vi "test1.vi"() -> ()   [LabVIEW 2014]
uses:
  <vilib>/Utility/sysdir.llb/System Directory Type.ctl
panel:
  in  "정규식":string
  out "이후 부분 문자열":string
  out "텍스트 2":string
  in  "오프셋(0)":i32=34
  in  "정규식 2":string
  out "이전 부분 문자열":string
  out "텍스트":string
  in  "오프셋(0) 2":i32=4
  out "연결된 문자열":string
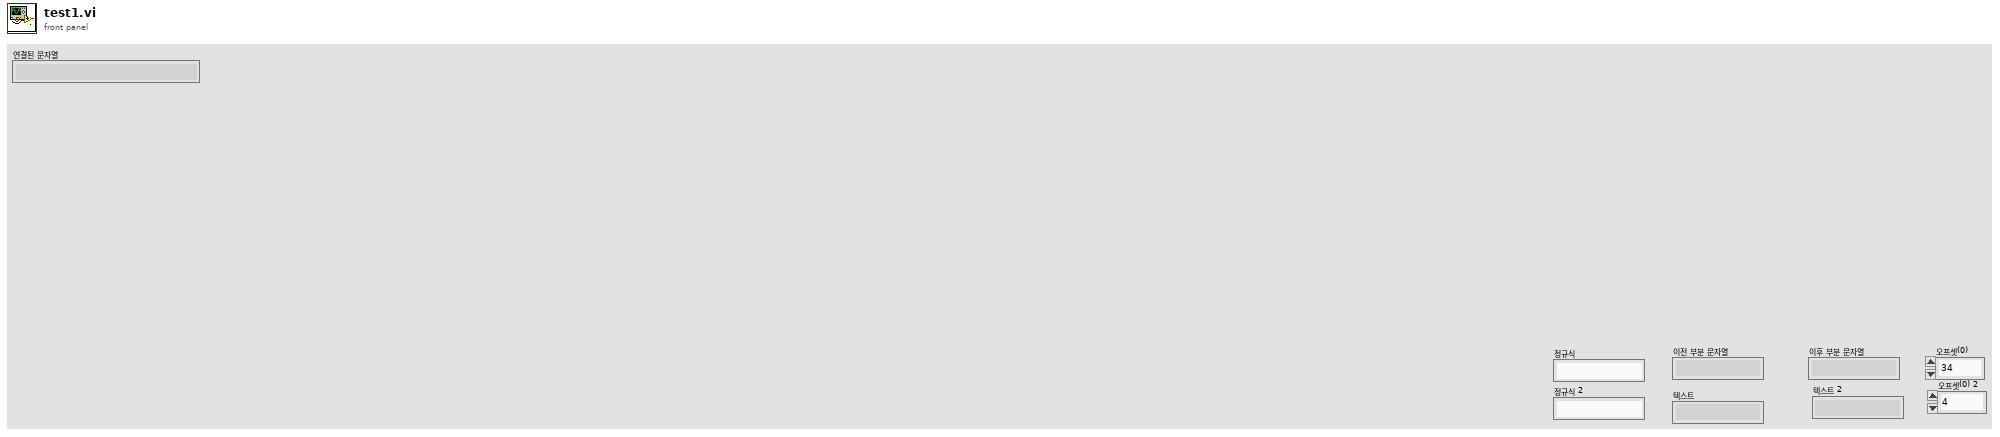
[diagram p1: front panel]
types:
  T1 = typedef "System Directory Type.ctl" = i32
  T2 = enum16{"open", "replace", "create", "open or create", "replace or create", "replace or create with confirmation"}
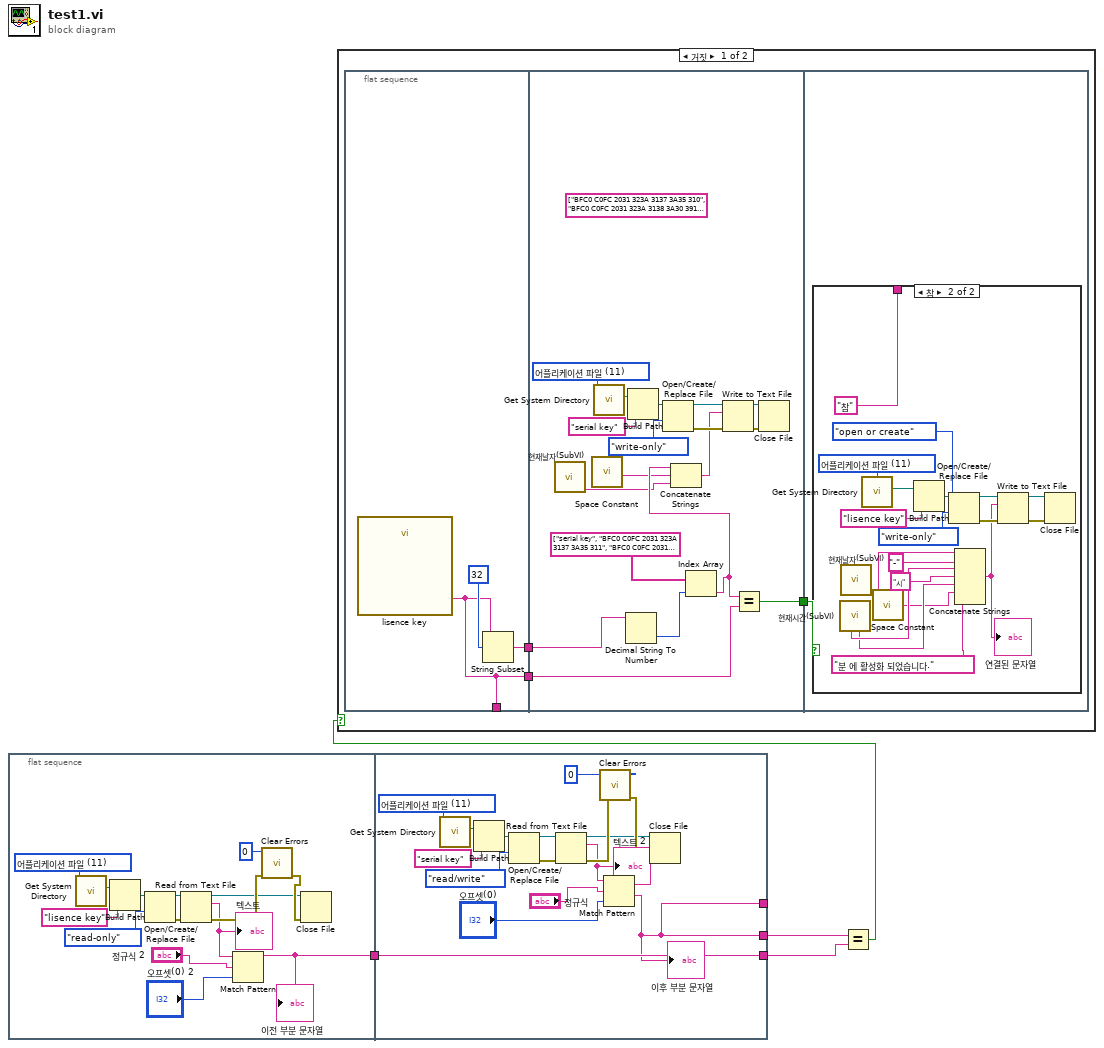
[diagram p0: block diagram]
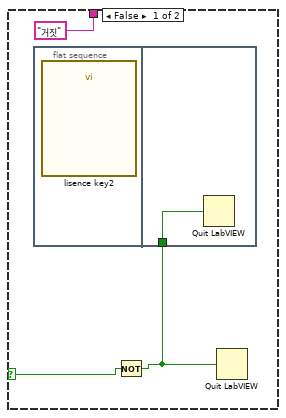
[diagram p2: hidden frame]
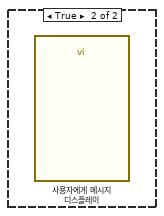
[diagram p3: hidden frame]
diagram:
  n1 = flat-sequence {
    tunnel: [w6] -> w4
    tunnel: [w22] -> w3
    tunnel: w4 -> [w22]
    tunnel: [w20] -> w2
    tunnel: [w20] -> _
    frame #0 {
      w9 = T1 11 items=["사용자 홈"=0, "사용자 데스크탑"=1, "사용자 문서"=2, "사용자 어플리케이션 데이터"=3, "사용자 환경"=4, "사용자 임시"=5, "퍼블릭 문서"=6, "퍼블릭 어플리케이션 데이터"=7, "퍼블릭 환경"=8, "퍼블릭 캐시"=13, "시스템 코어 라이브러리"=9, "시스템 설치된 라이브러리"=10, "어플리케이션 파일"=11, "부팅 볼륨 루트"=12] ("system directory type")
      n2 = call <vilib>:"Get System Directory.vi"("system directory type"=w9) -> ("system directory"=w8:path)  [unwired: 10 in]
      n3 = Build Path(base path=w8, name or relative path="lisence key" ("이름 또는 상대 경로")) -> (appended path=w7:path)
      n4 = Open/Create/Replace File(file path (use dialog)=w7, access (0:read/write)=enum16{"read/write", "read-only", "write-only"}."read-only" ("접근(0:읽기/쓰기)")) -> (refnum out=w13:refnum<file>, error out=w12:errorcluster)  [unwired: 4 in, 1 out]
      n5 = Read from Text File(file (use dialog)=w13, error in=w12) -> (refnum out=w14:refnum<file>, text=w15:string, error out=w17:errorcluster)  [unwired: 2 in, 1 out]
      "텍스트" <- w15
      n6 = Match Pattern(string=w15, regular expression="정규식 2", offset (0)="오프셋(0) 2") -> (before substring=w6:string)  [unwired: 3 out]
      "이전 부분 문자열" <- w6
      n7 = call <vilib>:"Clear Errors.vi"("error in (no error)"=w17, "specific error code to clear (0: all)"=0) -> ("error out"=w18:errorcluster)  [unwired: 4 in, 1 out]
      n8 = Close File(refnum=w14, error in=w18) -> ()  [unwired: 2 out]
    }
    frame #1 {
      w28 = T1 11 items=["사용자 홈"=0, "사용자 데스크탑"=1, "사용자 문서"=2, "사용자 어플리케이션 데이터"=3, "사용자 환경"=4, "사용자 임시"=5, "퍼블릭 문서"=6, "퍼블릭 어플리케이션 데이터"=7, "퍼블릭 환경"=8, "퍼블릭 캐시"=13, "시스템 코어 라이브러리"=9, "시스템 설치된 라이브러리"=10, "어플리케이션 파일"=11, "부팅 볼륨 루트"=12] ("system directory type")
      n9 = call <vilib>:"Get System Directory.vi"("system directory type"=w28) -> ("system directory"=w29:path)  [unwired: 10 in]
      n10 = Build Path(base path=w29, name or relative path="serial key" ("이름 또는 상대 경로")) -> (appended path=w30:path)
      n11 = Open/Create/Replace File(file path (use dialog)=w30, access (0:read/write)=enum16{"read/write", "read-only", "write-only"}."read/write" ("접근(0:읽기/쓰기)")) -> (refnum out=w24:refnum<file>, error out=w25:errorcluster)  [unwired: 4 in, 1 out]
      n12 = Read from Text File(file (use dialog)=w24, error in=w25) -> (refnum out=w23:refnum<file>, text=w31:string, error out=w33:errorcluster)  [unwired: 2 in, 1 out]
      "텍스트 2" <- w31
      n13 = call <vilib>:"Clear Errors.vi"("error in (no error)"=w33, "specific error code to clear (0: all)"=0) -> ("error out"=w34:errorcluster)  [unwired: 4 in, 1 out]
      n14 = Match Pattern(string=w31, regular expression="정규식", offset (0)="오프셋(0)") -> (after substring=w20:string)  [unwired: 3 out]
      "이후 부분 문자열" <- w20
      n15 = Close File(refnum=w23, error in=w34) -> ()  [unwired: 2 out]
    }
  }
  n16 = Equal?(x=w2, y=w3) -> (x = y?=w1:bool)
  n17 = case shown="거짓" w1 {
    frame False {
      n18 = flat-sequence {
        tunnel: [w40] -> w38
        tunnel: [w39] -> w37
        tunnel: [w39] -> _
        tunnel: w38 -> [w59]
        tunnel: [w56] -> w36
        tunnel: w37 -> [w57]
        tunnel: w36 -> [w60]
        frame #0 {
          n19 = call "lisence key"() -> ("lisence key"=w39:string)  [unwired: 17 in, 2 out]
          n20 = String Subset(string=w39, offset (0)=32 ("오프셋(0)")) -> (substring=w40:string)  [unwired: 1 in]
        }
        frame #1 {
          w49 = T1 11 items=["사용자 홈"=0, "사용자 데스크탑"=1, "사용자 문서"=2, "사용자 어플리케이션 데이터"=3, "사용자 환경"=4, "사용자 임시"=5, "퍼블릭 문서"=6, "퍼블릭 어플리케이션 데이터"=7, "퍼블릭 환경"=8, "퍼블릭 캐시"=13, "시스템 코어 라이브러리"=9, "시스템 설치된 라이브러리"=10, "어플리케이션 파일"=11, "부팅 볼륨 루트"=12] ("system directory type")
          (unwired) string[] ["BFC0 C0FC 2031 323A 3137 3A35 310", "BFC0 C0FC 2031 323A 3138 3A30 391", "BFC0 C0FC 2031 323A 3139 3A30 392", "BFC0 C0FC 2031 323A 3230 3A30 393", "BFC0 C0FC 2031 323A 3231 3A30 394", "BFC0 C0FC 2031 323A 3232 3A30 395", "BFC0 C0FC 2031 323A 3233 3A30 396", "BFC0 C0FC 2031 323A 3234 3A30 397", "BFC0 C0FC 2031 323A 3235 3A30 398", "BFC0 C0FC 2031 323A 3236 3A30 399", "BFC0 C0FC 2031 323A 3237 3A30 3910", "BFC0 C0FC 2031 323A 3238 3A30 3911", "BFC0 C0FC 2031 323A 3239 3A30 3912", "BFC0 C0FC 2031 323A 3036 3A33 3213", "BFC0 C0FC 2031 323A 3037 3A33 3214", "BFC0 C0FC 2031 323A 3038 3A33 3215", "BFC0 C0FC 2031 323A 3038 3A33 3216", "BFC0 C0FC 2031 323A 3039 3A33 3217", "BFC0 C0FC 2031 323A 3039 3A35 3018", "BFC0 C0FC 2031 323A 3130 3A35 3019", "BFC0 C0FC 2031 323A 3131 3A35 3120", "BFC0 C8C4 2031 313A 3536 3A33 3221", "BFC0 C8C4 2031 313A 3537 3A33 3222", "BFC0 C8C4 2031 313A 3538 3A33 3223", "BFC0 C8C4 2031 313A 3539 3A33 3224", "BFC0 C0FC 2031 323A 3030 3A33 3225", "BFC0 C0FC 2031 323A 3031 3A33 3226", "BFC0 C0FC 2031 323A 3032 3A33 3227", "BFC0 C0FC 2031 323A 3033 3A33 3228", "BFC0 C0FC 2031 323A 3034 3A33 3229", "BFC0 C0FC 2031 323A 3035 3A33 3230", "BFC0 C0FC 2031 323A 3036 3A33 3231", "BFC0 C0FC 2031 323A 3037 3A33 3232", "BFC0 C0FC 2031 323A 3038 3A33 3233"]
          n21 = call "현재날자(SubVI).vi"() -> ("월,일 을 문자열로"=w43:string)  [unwired: 5 in, 6 out]
          n22 = call <vilib>:"Space Constant.vi"() -> ("String"=w42:string)
          n23 = call <vilib>:"Get System Directory.vi"("system directory type"=w49) -> ("system directory"=w48:path)  [unwired: 10 in]
          n24 = Decimal String To Number(string=w59) -> (number=w58:i32)  [unwired: 2 in, 1 out]
          n25 = Build Path(base path=w48, name or relative path="serial key" ("이름 또는 상대 경로")) -> (appended path=w47:path)
          n26 = Open/Create/Replace File(file path (use dialog)=w47, access (0:read/write)=enum16{"read/write", "read-only", "write-only"}."write-only" ("접근(0:읽기/쓰기)")) -> (refnum out=w55:refnum<file>, error out=w54:errorcluster)  [unwired: 4 in, 1 out]
          n27 = Index Array(array=string[] ["serial key", "BFC0 C0FC 2031 323A 3137 3A35 311", "BFC0 C0FC 2031 323A 3138 3A30 392", "BFC0 C0FC 2031 323A 3139 3A30 393", "BFC0 C0FC 2031 323A 3230 3A30 394", "BFC0 C0FC 2031 323A 3231 3A30 395", "BFC0 C0FC 2031 323A 3232 3A30 396", "BFC0 C0FC 2031 323A 3233 3A30 397", "BFC0 C0FC 2031 323A 3234 3A30 398", "BFC0 C0FC 2031 323A 3235 3A30 399", "BFC0 C0FC 2031 323A 3236 3A30 3910", "BFC0 C0FC 2031 323A 3237 3A30 3911", "BFC0 C0FC 2031 323A 3238 3A30 3912", "BFC0 C0FC 2031 323A 3239 3A30 3913", "BFC0 C0FC 2031 323A 3036 3A33 3214", "BFC0 C0FC 2031 323A 3037 3A33 3215", "BFC0 C0FC 2031 323A 3038 3A33 3216", "BFC0 C0FC 2031 323A 3038 3A33 3217", "BFC0 C0FC 2031 323A 3039 3A33 3218", "BFC0 C0FC 2031 323A 3039 3A35 3019", "BFC0 C0FC 2031 323A 3130 3A35 3020", "BFC0 C0FC 2031 323A 3131 3A35 3121", "BFC0 C8C4 2031 313A 3536 3A33 3222", "BFC0 C8C4 2031 313A 3537 3A33 3223", "BFC0 C8C4 2031 313A 3538 3A33 3224", "BFC0 C8C4 2031 313A 3539 3A33 3225", "BFC0 C0FC 2031 323A 3030 3A33 3226", "BFC0 C0FC 2031 323A 3031 3A33 3227", "BFC0 C0FC 2031 323A 3032 3A33 3228", "BFC0 C0FC 2031 323A 3033 3A33 3229", "BFC0 C0FC 2031 323A 3034 3A33 3230", "BFC0 C0FC 2031 323A 3035 3A33 3231", "BFC0 C0FC 2031 323A 3036 3A33 3232", "BFC0 C0FC 2031 323A 3037 3A33 3233", "BFC0 C0FC 2031 323A 3038 3A33 3234", ""] ("출력 배열"), index=w58) -> (element=w44:string)
          n28 = Concatenate Strings(w44, w42, w43) -> (w46:string)
          n29 = Write to Text File(file (use dialog)=w55, text=w46, error in=w54) -> (refnum out=w52:refnum<file>, error out=w53:errorcluster)  [unwired: 1 in, 1 out]
          n30 = Equal?(x=w44, y=w57) -> (x = y?=w56:bool)
          n31 = Close File(refnum=w52, error in=w53) -> ()  [unwired: 2 out]
        }
        frame #2 {
          n32 = case shown="참" w60 {
            selector: w60 -> [w61 _]
            tunnel: ["거짓" "참"] -> _
            frame False {
              n33 = flat-sequence {
                tunnel: w62 -> [w64]
                frame #0 {
                  n34 = call "lisence key2"() -> ()  [unwired: 10 in, 2 out]
                }
                frame #1 {
                  n35 = Quit LabVIEW(quit? (T)=w64) -> ()
                }
              }
              n36 = Not(x=w61) -> (.not. x?=w62:bool)
              n37 = Quit LabVIEW(quit? (T)=w62) -> ()
            }
            frame True {
              w78 = T1 11 items=["사용자 홈"=0, "사용자 데스크탑"=1, "사용자 문서"=2, "사용자 어플리케이션 데이터"=3, "사용자 환경"=4, "사용자 임시"=5, "퍼블릭 문서"=6, "퍼블릭 어플리케이션 데이터"=7, "퍼블릭 환경"=8, "퍼블릭 캐시"=13, "시스템 코어 라이브러리"=9, "시스템 설치된 라이브러리"=10, "어플리케이션 파일"=11, "부팅 볼륨 루트"=12] ("system directory type")
              n38 = call "현재시간(SubVI).vi"() -> ("분 문자열"=w67:string, "시 문자열"=w69:string)  [unwired: 3 in, 7 out]
              n39 = call "현재날자(SubVI).vi"() -> ("월,일 을 문자열로"=w71:string)  [unwired: 5 in, 6 out]
              n40 = call <vilib>:"Get System Directory.vi"("system directory type"=w78) -> ("system directory"=w79:path)  [unwired: 10 in]
              n41 = call <vilib>:"Space Constant.vi"() -> ("String"=w66:string)
              n42 = Build Path(base path=w79, name or relative path="lisence key" ("이름 또는 상대 경로")) -> (appended path=w80:path)
              n43 = Open/Create/Replace File(file path (use dialog)=w80, operation (0:open)=T2."open or create" ("동작(0:open)"), access (0:read/write)=enum16{"read/write", "read-only", "write-only"}."write-only" ("접근(0:읽기/쓰기)")) -> (refnum out=w76:refnum<file>, error out=w74:errorcluster)  [unwired: 3 in, 1 out]
              n44 = Concatenate Strings(w71, "-", w69, "시", w67, w66, "분 에 활성화 되었습니다.") -> (w72:string)
              "연결된 문자열" <- w72
              n45 = Write to Text File(file (use dialog)=w76, text=w72, error in=w74) -> (refnum out=w77:refnum<file>, error out=w73:errorcluster)  [unwired: 1 in, 1 out]
              n46 = Close File(refnum=w77, error in=w73) -> ()  [unwired: 2 out]
            }
          }
        }
      }
    }
    frame True {
      n47 = call "사용자에게 메시지 디스플레이"() -> ()  [unwired: 10 in, 2 out]
    }
  }
